vi "Execute.vi"(8 "error in (no error)":errorcluster, 10 "System In":refnum<class "abs_System.lvclass">, 11 "Node in":refnum<class "Succeed.lvclass">) -> (0 "error out":errorcluster, 1 "Status":T1, 2 "System Out":refnum<class "abs_System.lvclass">, 3 "Node out":refnum<class "Succeed.lvclass">)   [LabVIEW 2021, in "BT.lvlib" / "Succeed.lvclass"]
uses:
  Succeed.lvclass
  abs_Node/Status.ctl
  abs_System/abs_System.lvclass
  abs_Decorator/abs_Decorator.lvclass
  abs_Node/abs_Node.lvclass
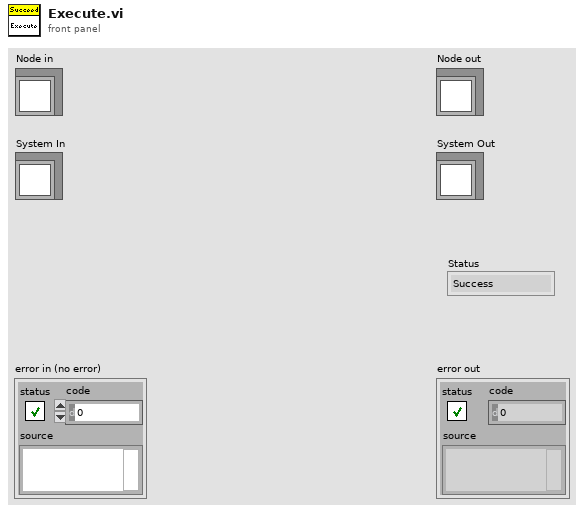
[diagram p1: front panel]
types:
  T1 = typedef "BT.lvlib/abs_Node.lvclass/Status.ctl" = enum16{"Success", "Failure", "Running"}
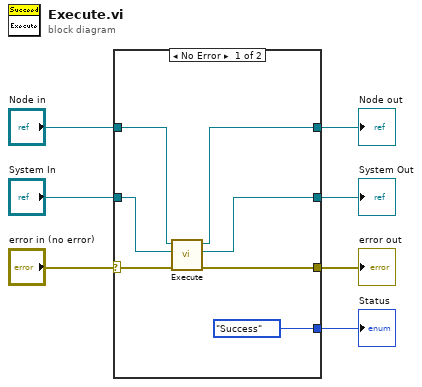
[diagram p0: block diagram]
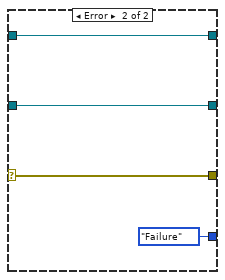
[diagram p2: hidden frame]
diagram:
  n1 = case shown="No Error" "error in (no error)" {
    selector: "error in (no error)" -> [w11 w16]
    tunnel: [w14 w16] -> w7
    tunnel: [w13 w17] -> w6
    tunnel: [w12 w18] -> w5
    tunnel: "System In" -> [w10 w17]
    tunnel: "Node in" -> [w9 w18]
    tunnel: [Status."Success" ("Status") Status."Failure" ("Status")] -> w1
    frame No Error {
      n2 = call-parent "Execute.vi"("error in (no error)"=w11, "System In"=w10, "Node in"=w9) -> ("error out"=w14:errorcluster, "System Out"=w13:refnum<class "abs_System.lvclass">, "Node out"=w12:refnum<class "Succeed.lvclass">)  [unwired: 5 in, 1 out]
    }
    frame Error {
    }
  }
  "error out" <- w7
  "Node out" <- w5
  "Status" <- w1
  "System Out" <- w6
